vi "Add LabVIEW Error.vi"(8 "error in (no error)":errorcluster, 10 "LabVIEW Error":errorcluster, 11 "Alarm Handler Actor in":refnum<class "Error Handler Actor.lvclass">) -> (0 "error out":errorcluster, 3 "Alarm Handler Actor out":refnum<class "Error Handler Actor.lvclass">)   [LabVIEW 2021, in "Error Handler Actor.lvclass"]
uses:
  Error Handler Actor.lvclass
  Error Handler Actor.lvclass/Error Handler Actor.ctl
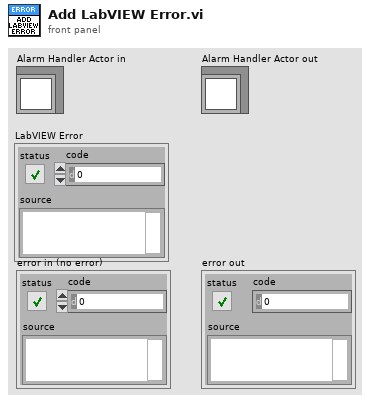
[diagram p1: front panel]
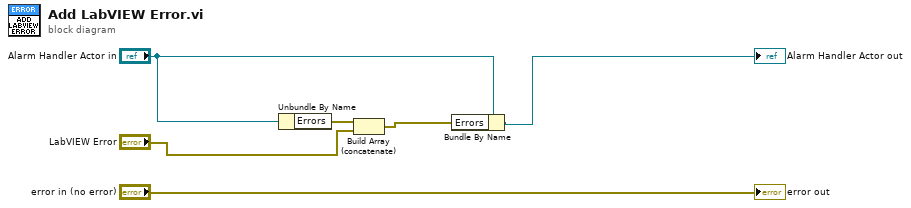
[diagram p0: block diagram]
diagram:
  n1 = Unbundle By Name("Alarm Handler Actor in") -> ("Errors"=w6:errorcluster[])
  n2 = Build Array (concatenate)(w6, "LabVIEW Error") -> (w3:errorcluster[])
  n3 = Bundle By Name(cluster="Alarm Handler Actor in", "Errors"=w3) -> (→"Alarm Handler Actor out":refnum<class "Error Handler Actor.lvclass">)
  "error out" <- "error in (no error)"
